vi "Thorlabs EVOA 1550 power control.vi"() -> ()   [LabVIEW 2018]
panel:
  in  "clear 2":bool
  out "Monitior Power (channel 4)":dbl(graph)=0.007796702841283286
  in  "clear":bool
  out "Photodetector Power (channel 3)":dbl(graph)=0.007796702841283286
  in  "Modulation voltage":dbl(slide) scale=0.0..5.0
  in  "stop":bool
  # "Output"
  # "EVOA Monitor"
  # "EVOA # 1"
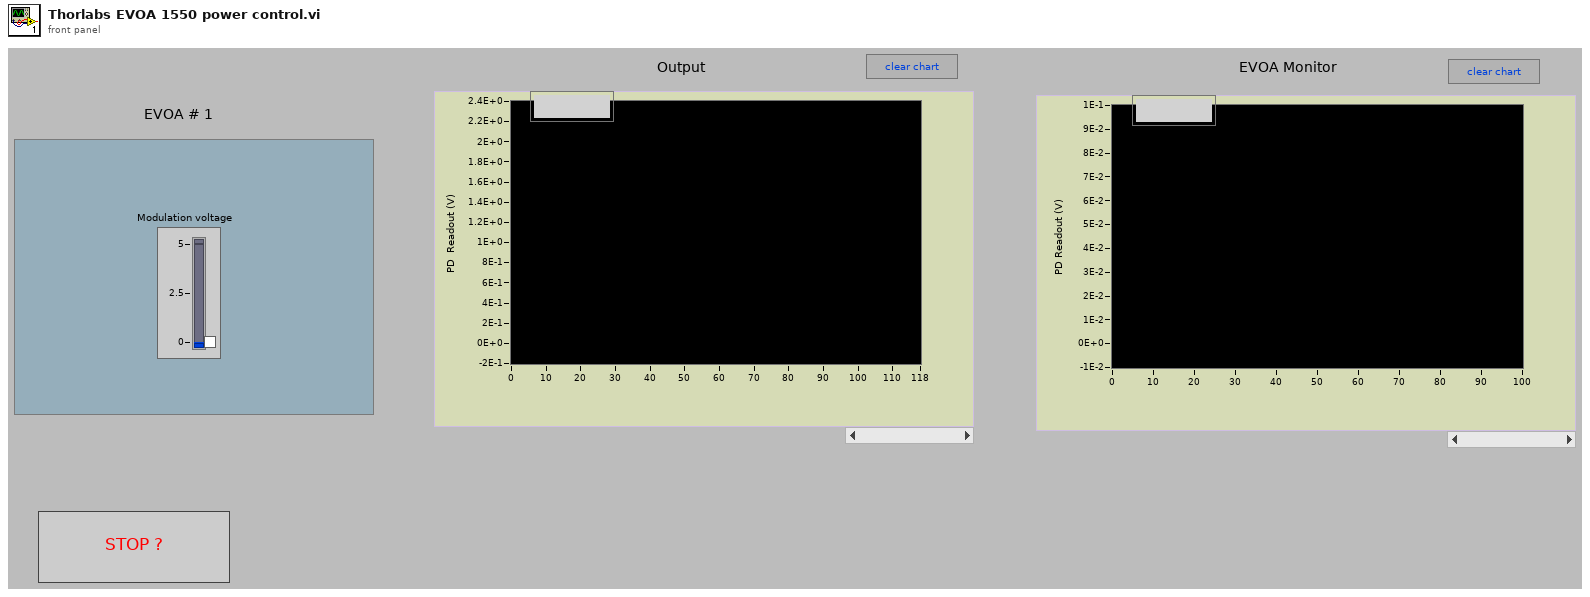
[diagram p1: front panel]
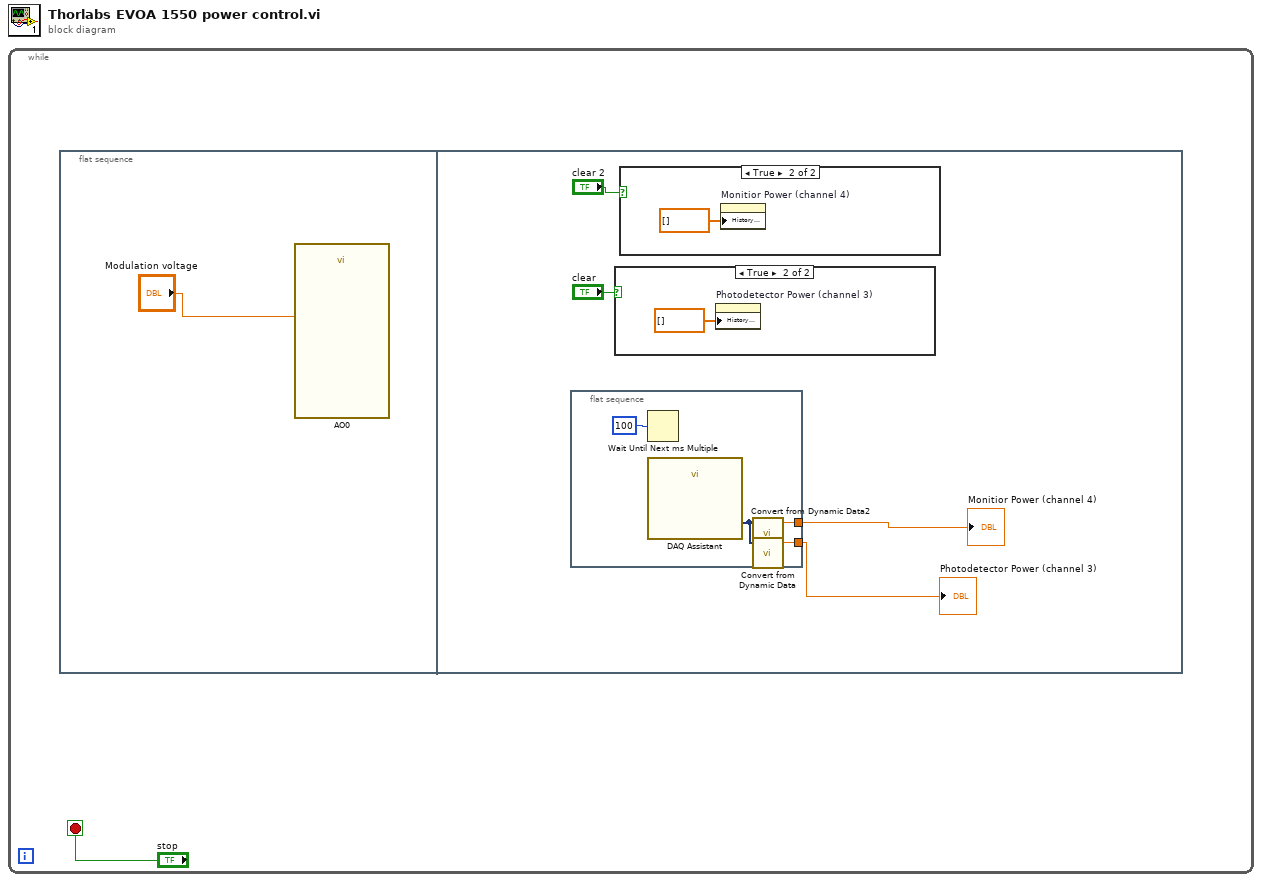
[diagram p0: block diagram]
diagram:
  n1 = while {
    stop <- "stop" stop-if-true
    n2 = flat-sequence {
      frame #0 {
        n3 = call "AO0"("data"="Modulation voltage") -> ()  [unwired: 17 in, 2 out]
      }
      frame #1 {
        n4 = flat-sequence {
          tunnel: [w11] -> w3
          tunnel: [w10] -> w4
          frame #0 {
            n5 = Wait Until Next ms Multiple(millisecond multiple=u32 100 ("milliseconds to wait")) -> ()  [unwired: 1 out]
            n6 = call "DAQ Assistant"() -> ("data"=w9:dynamicdata)  [unwired: 17 in, 2 out]
            n7 = call "Convert from Dynamic Data2"("Dynamic Data Type"=w9) -> ("Scalar"=w10:dbl)  [unwired: 3 in]
            n8 = call "Convert from Dynamic Data"("Dynamic Data Type"=w9) -> ("Scalar"=w11:dbl)  [unwired: 3 in]
          }
        }
        n9 = case shown="True" "clear" {
          frame False {
          }
          frame True {
            n10 = property on="Photodetector Power (channel 3)" class="WFChart (strict)"("History Data"=dbl[] []) -> ()  [unwired: 2 in, 2 out]
          }
        }
        n11 = case shown="True" "clear 2" {
          frame False {
          }
          frame True {
            n12 = property on="Monitior Power (channel 4)" class="WFChart (strict)"("History Data"=dbl[] []) -> ()  [unwired: 2 in, 2 out]
          }
        }
        "Photodetector Power (channel 3)" <- w3
        "Monitior Power (channel 4)" <- w4
      }
    }
  }
